vi "test1_fromALCN.vi"() -> ()   [LabVIEW 2009]
panel:
  out "Array 3":i32[](array[numeric])
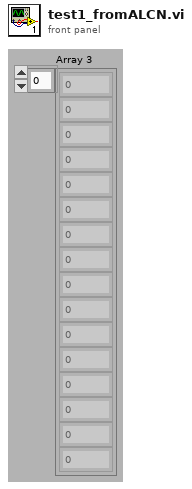
[diagram p1: front panel]
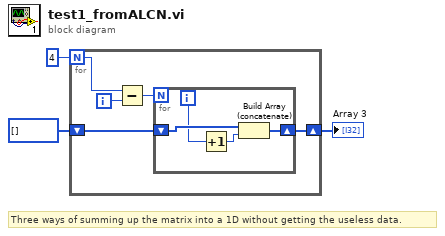
[diagram p0: block diagram]
diagram:
  # "Three ways of summing up the matrix into a 1D without getting the useless data."
  n1 = for {
    N: 4 -> [w8]
    shift-right: [w4] -> w3
    shift-left: i32[] [] -> [w5]
    i -> [w7]
    n2 = Subtract(x=w8, y=w7) -> (x-y=w6:i32)
    n3 = for {
      N: w6 -> [_]
      shift-right: [w11] -> w4
      shift-left: w5 -> [w12]
      i -> [w10]
      n4 = Increment(x=w10) -> (x+1=w9:i32)
      n5 = Build Array (concatenate)(w12, w9) -> (w11:i32[])
    }
  }
  "Array 3" <- w3
